vi "Remove Self Secion.vi"(10 "Section Name":string, 11 "Section Node Data":string[](array[string])) -> (3 "Updated Section Node":string[](array[string]))   [LabVIEW 2025]
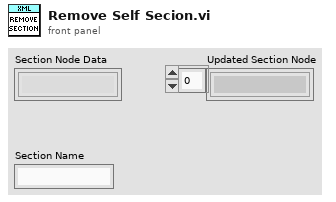
[diagram p1: front panel]
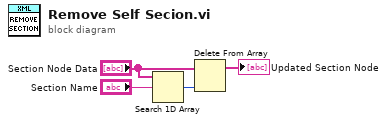
[diagram p0: block diagram]
diagram:
  n1 = Search 1D Array(1D array="Section Node Data", element="Section Name") -> (index of element=w3:i32)  [unwired: 1 in]
  n2 = Delete From Array(array="Section Node Data", index=w3) -> (array with subset deleted=→"Updated Section Node":string[])  [unwired: 1 in, 1 out]
